vi "Supported Smart Syntax Representation.vi"(0 "For Loop in":refnum<class "While Loop.lvclass">, 11 "error in (no error)":errorcluster) -> (4 "For Loop out":refnum<class "While Loop.lvclass">, 6 "Smart Syntax Representation List":string[](array[string]), 15 "error out":errorcluster)   [LabVIEW 2016, in "While Loop.lvclass"]
uses:
  While Loop.lvclass
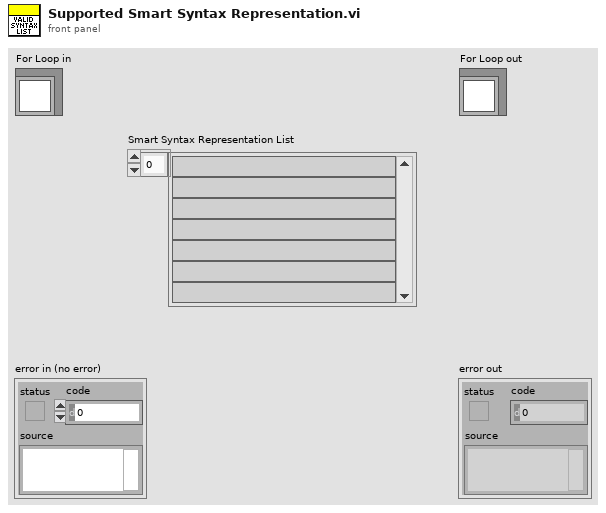
[diagram p1: front panel]
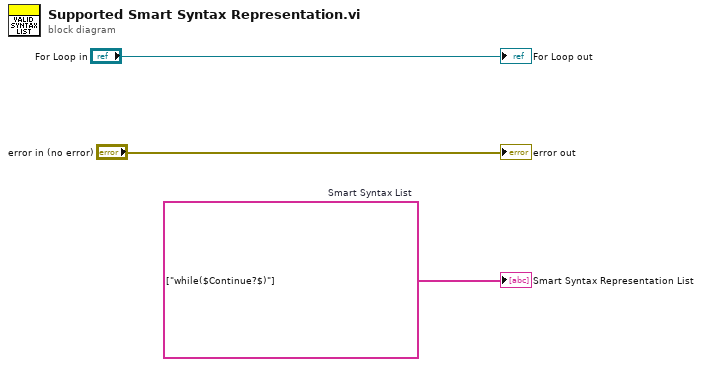
[diagram p0: block diagram]
diagram:
  w1 = string[] ["while($Continue?$)"]  # Smart Syntax List
  "error out" <- "error in (no error)"
  "For Loop out" <- "For Loop in"
  "Smart Syntax Representation List" <- w1
